vi "writelog.vi"(7 "Date":string, 10 "Message":string, 11 "file path (use dialog)":path) -> ()   [LabVIEW 2014]
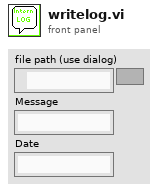
[diagram p1: front panel]
types:
  T1 = enum16{"open", "replace", "create", "open or create", "replace or create", "replace or create with confirmation"}
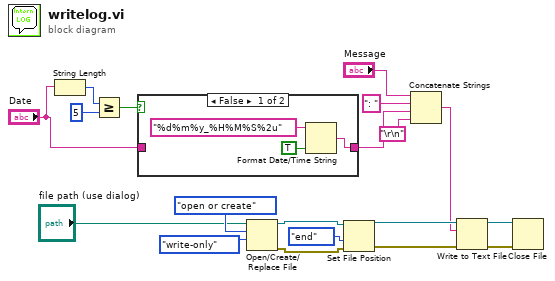
[diagram p0: block diagram]
diagram:
  n1 = String Length(string="Date") -> (length=w6:i32)
  n2 = Greater Or Equal?(x=w6, y=5) -> (x >= y?=w4:bool)
  n3 = case shown="False" w4 {
    tunnel: "Date" -> [_ w23]
    tunnel: [w20 w23] -> w2
    frame False {
      n4 = Format Date/Time String(time format string (%c)="%d%m%y_%H%M%S%2u", UTC format=TRUE) -> (date/time string=w20:string)  [unwired: 1 in]
    }
    frame True {
    }
  }
  n5 = Open/Create/Replace File(file path (use dialog)="file path (use dialog)", operation (0:open)=T1."open or create", access (0:read/write)=enum16{"read/write", "read-only", "write-only"}."write-only") -> (refnum out=w17:refnum<file>, error out=w16:errorcluster)  [unwired: 3 in, 1 out]
  n6 = Set File Position(refnum=w17, from (0:start)=enum16{"start", "end", "current"}."end", error in=w16) -> (refnum out=w14:refnum<file>, error out=w13:errorcluster)  [unwired: 1 in]
  n7 = Concatenate Strings("Message", ": " ("string"), w2, "\r\n") -> (w9:string)
  n8 = Write to Text File(file (use dialog)=w14, text=w9, error in=w13) -> (refnum out=w12:refnum<file>, error out=w11:errorcluster)  [unwired: 1 in, 1 out]
  n9 = Close File(refnum=w12, error in=w11) -> ()  [unwired: 2 out]
